vi "Lock Publication.vi"(4 "Return Error Transport":refnum<class "ITransport.lvclass">, 6 "Publisher ID":string, 7 "PublicationPolicy":refnum<class "IPublicationPolicy.lvclass">, 8 "error in (no error)":errorcluster, 9 "Datum Type":variant, 10 "Datum Name":string, 11 "IMediator In":refnum<class "IMediator.lvclass">) -> (0 "error out":errorcluster, 3 "IMediator Out":refnum<class "IMediator.lvclass">)   [LabVIEW 2017, in "IMediator.lvlib" / "IMediator.lvclass"]
doc: "<License>\nCopyright © 2017 Composed Systems, LLC | All rights reserved\nwww.composed.io\n\nAuthor: Ethan Stern <ethan.stern@composed.io>\n\nThis software is provided \"AS IS\" WITHOUT WARRANTIES, either express or implied, AND IS FOR EDUCATIONAL PURPOSES ONLY.\n</License>"
uses:
  IMediator.lvclass
  gpm_packages/@cs/transport/Source/ITransport/ITransport.lvclass
  IPublicationPolicy/IPublicationPolicy.lvclass
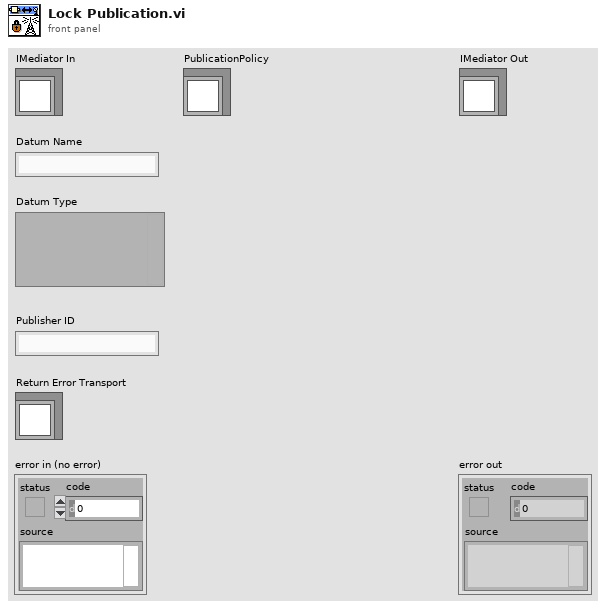
[diagram p1: front panel]
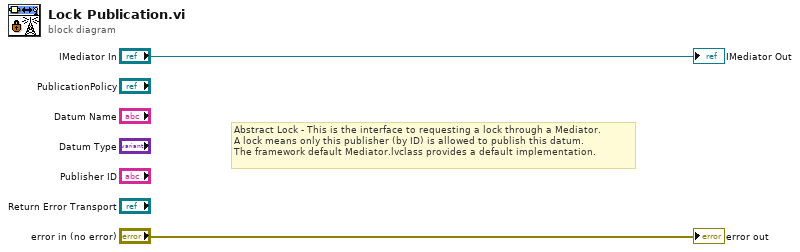
[diagram p0: block diagram]
diagram:
  # "Abstract Lock - This is the interface to requesting a lock through a Mediator.\nA lock means only this publisher (by ID) is allowed to publish this datum.\nThe framework default Mediator.lvclass provides a default implementation."
  "error out" <- "error in (no error)"
  "IMediator Out" <- "IMediator In"
